vi "G_Posiciones_Variables.vi"() -> ()   [LabVIEW 2020]
panel:
  in  "Posiciones Variables":T1={"Desmenuzadora (x)"=24, "Desmenuzadora (y)"=180, "Aspa (x)"=49, "Aspa (y)"=231, "Masa elevador (x)"=253, "Masa elevador (y) "=209, "Galletas Molde (x)"=852, "Galletas Molde (y)"=169, "Galletas Horno (x) "=1068, "Galletas Horno (y) "=361, "Galletas Enfria (x) "=144, "Galletas Enfria (y) "=558}
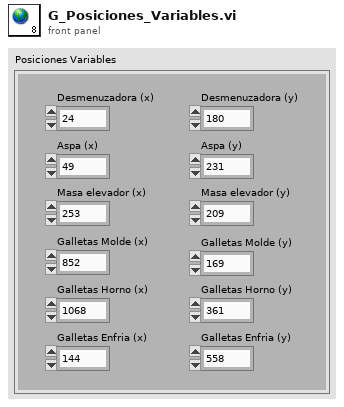
[diagram p1: front panel]
types:
  T1 = cluster{"Desmenuzadora (x)":i32, "Desmenuzadora (y)":i32, "Aspa (x)":i32, "Aspa (y)":i32, "Masa elevador (x)":i32, "Masa elevador (y) ":i32, "Galletas Molde (x)":i32, "Galletas Molde (y)":i32, "Galletas Horno (x) ":i32, "Galletas Horno (y) ":i32, "Galletas Enfria (x) ":i32, "Galletas Enfria (y) ":i32}
diagram:
